vi "Open Gateway wrapper.vi"(8 "error in (no error)":errorcluster caption="错误输入（无错误）", 9 "iLen":i32=1024, 11 "dwDevIndex":u32) -> (0 "error out":errorcluster caption="错误输出", 2 "subNodeIdlist out":u32[](array[numeric]), 3 "function return":i32, 5 "pdCanBtr out":u32)   [LabVIEW 2016, in "UISimCanFunc_wrapper.lvlib"]
doc: "_declspec (dllexport) DWORD OpenGateway_wrapper(DWORD dwDevIndex, DWORD subNodeIdlist[], int iLen, PDWORD pdCanBtr);"
uses:
  <userlib>/UISimCanFunc_wrapper/UISimCanFunc_wrapper.lvlib
  <userlib>/UISimCanFunc_wrapper/UISimCanFunc_wrapper.dll
panel:
  in  "pdCanBtr":u32
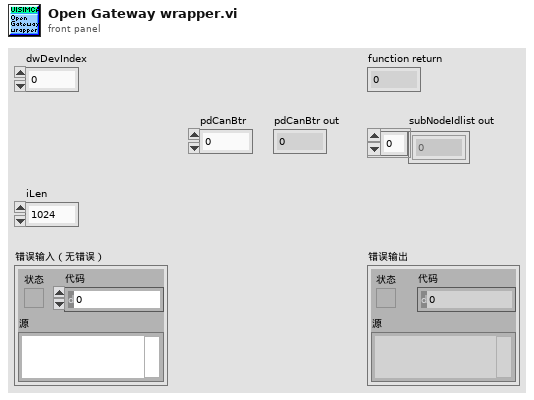
[diagram p1: front panel]
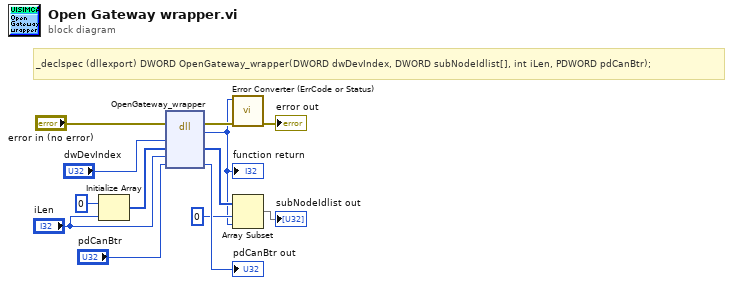
[diagram p0: block diagram]
diagram:
  # "_declspec (dllexport) DWORD OpenGateway_wrapper(DWORD dwDevIndex, DWORD subNodeIdlist[], int iLen, PDWORD pdCanBtr);"
  n1 = Initialize Array(u32 0 ("元素"), "iLen") -> (w7:u32[])
  n2 = dll-call lib="C:/Program Files (x86)/National Instruments/LabVIEW 2016/user.lib/UISimCanFunc_wrapper/UISimCanFunc_wrapper.*" fn="OpenGateway_wrapper"(error in="error in (no error)", "dwDevIndex"="dwDevIndex", "subNodeIdlist"=w7, "iLen"="iLen", "pdCanBtr"="pdCanBtr") -> (error out=w9:errorcluster, "返回类型"=w2:i32, "subNodeIdlist"=w4:u32[], "pdCanBtr"=→"pdCanBtr out":u32)  [unwired: 4 in, 1 out]
  "function return" <- w2
  n3 = call <userlib>:"Error Converter (ErrCode or Status).vi"("error in (no error)"=w9, "error code"=w2) -> ("error out"=→"error out":errorcluster)  [unwired: 9 in]
  n4 = Array Subset(array=w4, index=0 ("索引"), length=w2) -> (→"subNodeIdlist out":u32[])
